vi "missionLocation.vi"(8 "Error In":errorcluster, 11 "GenericMission in":refnum<class "GenericMission.lvclass">) -> (0 "Error Out":errorcluster, 2 "element":T1 {"North" format="%#_10f"; "East" format="%#_8f"}, 3 "GenericMission out":refnum<class "GenericMission.lvclass">)   [LabVIEW 2013, in "GenericMission.lvclass"]
doc: "Get the key location for the mission for use on maps, etc. Should not need to be overriden by child classes."
uses:
  GenericMission.lvclass
  Data/TypeDefs/UTM Location.ctl
  GenericMission.lvclass/GenericMission.ctl
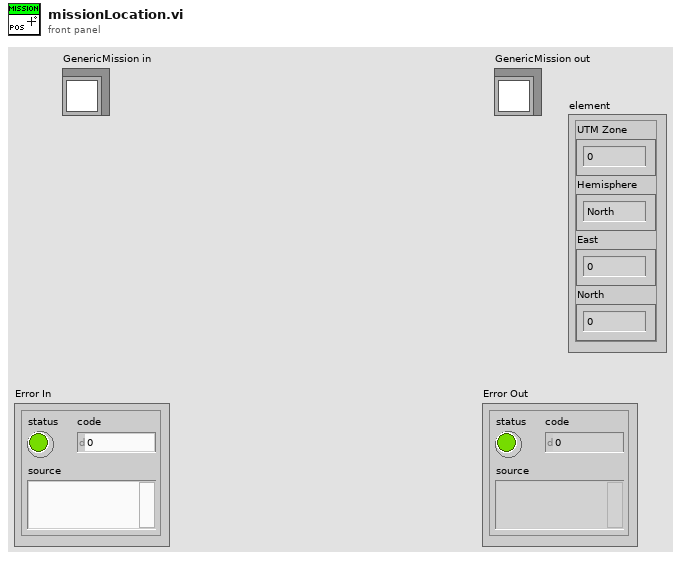
[diagram p1: front panel]
types:
  T1 = typedef "UTM Location.ctl" = cluster{"UTM Zone":dbl, "Hemisphere":enum16{"North", "South"}, "East":dbl, "North":dbl}
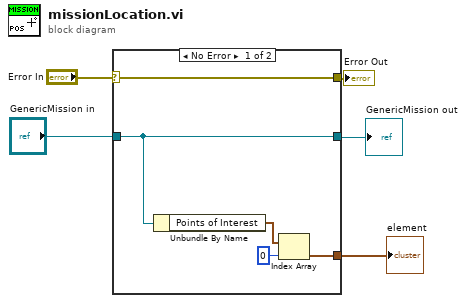
[diagram p0: block diagram]
diagram:
  n1 = case shown="No Error" "Error In" {
    selector: "Error In" -> [w10 w11]
    tunnel: [w10 w11] -> w4
    tunnel: "GenericMission in" -> [w9 w12]
    tunnel: [w9 w12] -> w2
    tunnel: [w6 _] -> w1
    frame No Error {
      n2 = Unbundle By Name(w9) -> ("Points of Interest"=w8:T1[])
      n3 = Index Array(array=w8, index=0) -> (element=w6:T1)
    }
    frame Error {
    }
  }
  "Error Out" <- w4
  "GenericMission out" <- w2
  "element" <- w1
